vi "to string.vi"(8 "error in":errorcluster, 11 "UI Reference configuration in":refnum<class "UI Reference configuration.lvclass">) -> (0 "error out":errorcluster, 1 "data":string, 2 "version":string, 3 "UI Reference configuration out":refnum<class "UI Reference configuration.lvclass">)   [LabVIEW 2013, in "UI Reference configuration.lvclass"]
doc: "Provides an interface for saving a module configuration to a file or other serialized data source. It is recommended that all children of this class store data in two sets--data required for its own initialization, and any data required for parent initialization--and that each implementation uses the <b>Call Parent Method</b> primitive to serialize parent information."
uses:
  UI Reference configuration.lvclass
  <vilib>/NI/Tag Bus Module Framework/module configuration/TBM module configuration.lvclass
  UI Reference configuration.lvclass/UI Reference configuration.ctl
  <vilib>/NI/Tag Bus Module Framework/root configuration/TBM configuration.lvclass
  <vilib>/NI/Tag Bus Module Framework/channel/TBM channel.lvclass
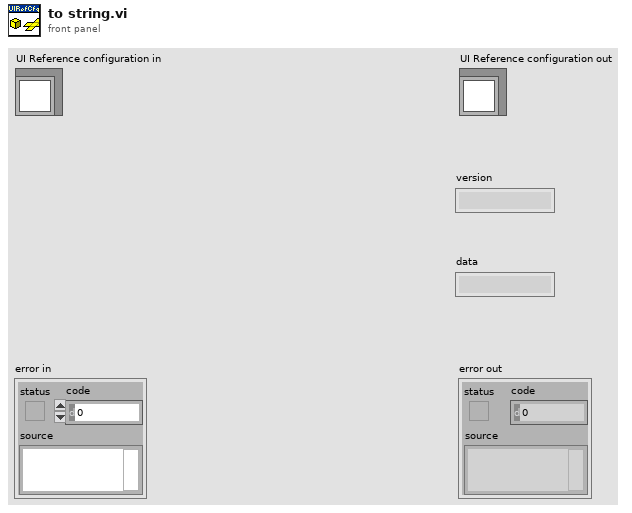
[diagram p1: front panel]
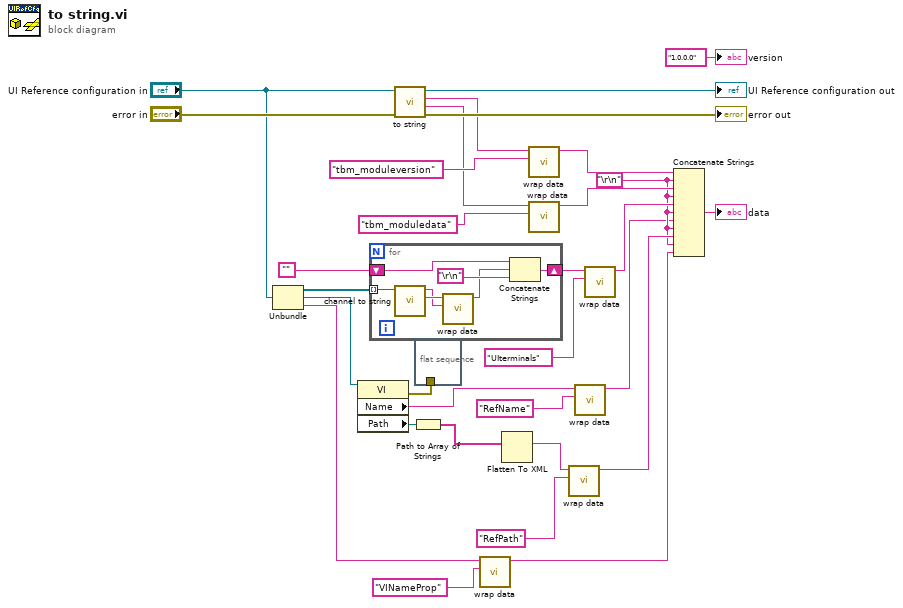
[diagram p0: block diagram]
diagram:
  w6 = "\r\n"
  n1 = Unbundle("UI Reference configuration in") -> (w18:refnum<class "TBM channel.lvclass">[], w9:refnum<vi>, w13:string)
  n2 = property class="VI"(reference=w9) -> (error out=w1:errorcluster, "Name"=w2:string, "Path"=w8:path)  [unwired: 1 in, 1 out]
  n3 = for {
    tunnel: w18 -> [w38] mode=indexing
    shift-right: [w34] -> w16
    shift-left: "" -> [w33]
    n4 = call <vilib>:"channel to string.vi"("channel in"=w38) -> ("channel data"=w37:string, "identifier"=w36:string)  [unwired: 9 in]
    n5 = call <vilib>:"wrap data.vi"("identifier"=w36, "data to wrap"=w37) -> ("wrapped data"=w32:string)  [unwired: 9 in]
    n6 = Concatenate Strings(w33, w32, "\r\n") -> (w34:string)
  }
  n7 = call-parent "to string.vi"("error in"="error in", "module configuration in"="UI Reference configuration in") -> ("error out"=→"error out":errorcluster, "data"=w23:string, "version"=w24:string, "module configuration out"=→"UI Reference configuration out":refnum<class "UI Reference configuration.lvclass">)  [unwired: 6 in]
  n8 = Path to Array of Strings(0:w8) -> (2:w4:string[])  [unwired: 1 out]
  n9 = flat-sequence {
    tunnel: w1 -> [_]
    frame #0 {
    }
  }
  n10 = call <vilib>:"wrap data.vi"("identifier"="VINameProp" ("additional identifier"), "data to wrap"=w13) -> ("wrapped data"=w12:string)  [unwired: 9 in]
  n11 = Flatten To XML(anything=w4) -> (xml string=w3:string)
  n12 = call <vilib>:"wrap data.vi"("identifier"="tbm_moduleversion" ("additional identifier"), "data to wrap"=w24) -> ("wrapped data"=w26:string)  [unwired: 9 in]
  n13 = call <vilib>:"wrap data.vi"("identifier"="tbm_moduledata" ("additional identifier"), "data to wrap"=w23) -> ("wrapped data"=w25:string)  [unwired: 9 in]
  n14 = call <vilib>:"wrap data.vi"("identifier"="RefPath" ("additional identifier"), "data to wrap"=w3) -> ("wrapped data"=w11:string)  [unwired: 9 in]
  n15 = call <vilib>:"wrap data.vi"("identifier"="RefName" ("additional identifier"), "data to wrap"=w2) -> ("wrapped data"=w5:string)  [unwired: 9 in]
  n16 = call <vilib>:"wrap data.vi"("identifier"="UIterminals" ("additional identifier"), "data to wrap"=w16) -> ("wrapped data"=w20:string)  [unwired: 9 in]
  n17 = Concatenate Strings(w26, w6, w25, w6, w20, w6, w5, w6, w11, w6, w12) -> (→"data":string)
  "version" <- "1.0.0.0" ("version")
